vi "ReadWrite Label.vi"(5 "Mode":T13, 6 "ScheduledSDI":bool, 7 "Iteration":i32, 8 "error in (no error)":errorcluster, 10 "FIFOs In":T1, 11 "Label In":T2 {"Words"."Param Setting"."Num Bits" min=1 max=32; "Words"."Param Setting"."Start Bit" min=8 max=31; "Words"."Block Data Refs"."Data Reference" format="%.0x"; "Label" format="%.0o"}) -> (0 "error out":errorcluster, 2 "FIFOs Out":T1, 3 "Label Out":T2 {"Words"."Param Setting"."Num Bits" min=1 max=32; "Words"."Param Setting"."Start Bit" min=8 max=31; "Words"."Block Data Refs"."Data Reference" format="%.0x"; "Label" format="%.0o"})   [LabVIEW 2012, in "AIT 429 Custom Device.lvlib"]
uses:
  AIT 429 Custom Device.lvlib
  RT Controls/ReadWrite Selector.ctl
  Controls and Global/Label.ctl
  Controls and Global/transferPeriod.ctl
  <vilib>/NI Veristand/Custom Device API/Data Reference.ctl
  <vilib>/NI Veristand/Custom Device API/Custom Device API.lvlib
  <vilib>/NI Veristand/Custom Device API/Block Data Reference.ctl
  Controls and Global/Start Bit.ctl
  Controls and Global/Number of Bits.ctl
  RT Controls/RT Label Settings.ctl
  RT Controls/FIFO.ctl
  RT Controls/Driver Data.ctl
  RT Controls/RT Param Setting.ctl
  RT Controls/RT Word Settings.ctl
  Controls and Global/TransferType.ctl
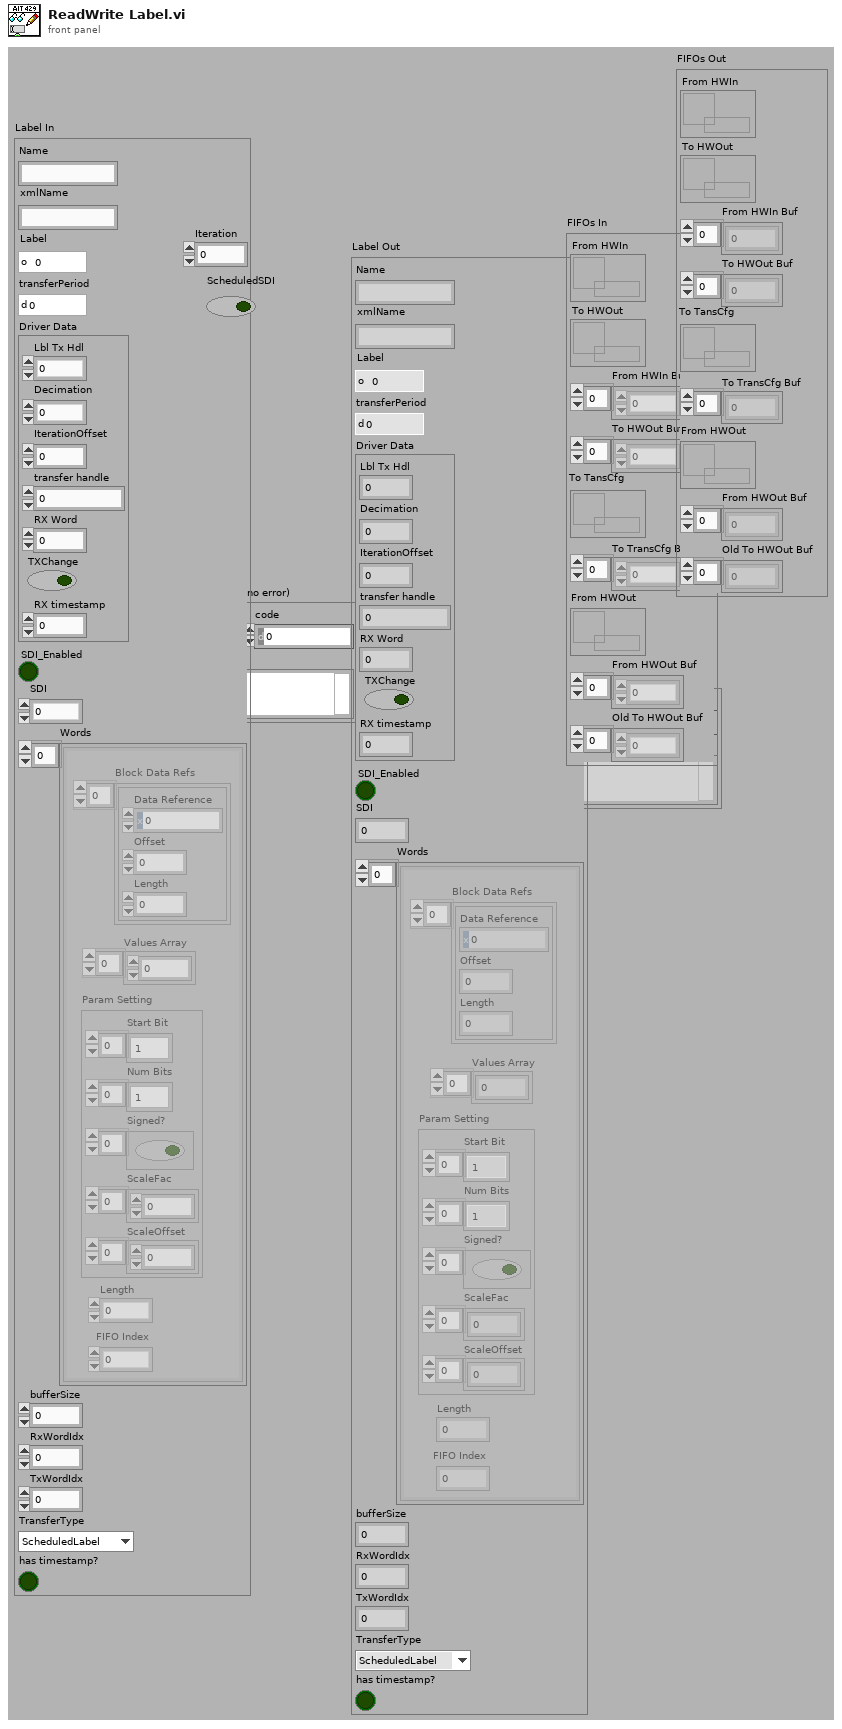
[diagram p1: front panel]
types:
  T1 = typedef "AIT 429 Custom Device.lvlib/FIFO.ctl" = cluster{"From HWIn":refnum<k33>, "To HWOut":refnum<k33>, "From HWIn Buf":dbl[], "To HWOut Buf":dbl[], "To TansCfg":refnum<k33>, "To TransCfg Buf":dbl[], "From HWOut":refnum<k33>, "From HWOut Buf":dbl[], "Old To HWOut Buf":dbl[]}
  T2 = typedef "AIT 429 Custom Device.lvlib/RT Label Settings.ctl" = cluster{"Name":string, "xmlName":string, "Label":T3, "transferPeriod":T4, "Driver Data":T5, "SDI_Enabled":bool, "SDI":u8, "Words":T6[], "bufferSize":u32, "RxWordIdx":i32, "TxWordIdx":i32, "TransferType":T12, "has timestamp?":bool}
  T3 = typedef "AIT 429 Custom Device.lvlib/Label.ctl" = u8
  T4 = typedef "AIT 429 Custom Device.lvlib/transferPeriod.ctl" = u32
  T5 = typedef "AIT 429 Custom Device.lvlib/Driver Data.ctl" = cluster{"Lbl Tx Hdl":u32, "Decimation":i32, "IterationOffset":i32, "transfer handle":u32, "RX Word":u32, "TXChange":bool, "RX timestamp":dbl}
  T6 = typedef "AIT 429 Custom Device.lvlib/RT Word Settings.ctl" = cluster{"Block Data Refs":T7[], "Values Array":dbl[], "Length":i32, "FIFO Index":i32, "Param Setting":T9}
  T7 = typedef "Custom Device API.lvlib/Block Data Reference.ctl" = cluster{"Data Reference":T8, "Offset":i32, "Length":i32}
  T8 = typedef "Custom Device API.lvlib/Data Reference.ctl" = i32
  T9 = typedef "AIT 429 Custom Device.lvlib/Rt Param Setting.ctl" = cluster{"Start Bit":T10[], "Num Bits":T11[], "Signed?":bool[], "ScaleFac":dbl[], "ScaleOffset":dbl[]}
  T10 = typedef "AIT 429 Custom Device.lvlib/Start Bit.ctl" = i32
  T11 = typedef "AIT 429 Custom Device.lvlib/Number of Bits.ctl" = i32
  T12 = typedef "AIT 429 Custom Device.lvlib/TransferType.ctl" = enum16{"ScheduledLabel", "Acyclic", "Block", "Strobe"}
  T13 = typedef "AIT 429 Custom Device.lvlib/ReadWrite Selector.ctl" = enum16{"Inline Read", "Inline Write", "Async HWIn", "Async HWOut"}
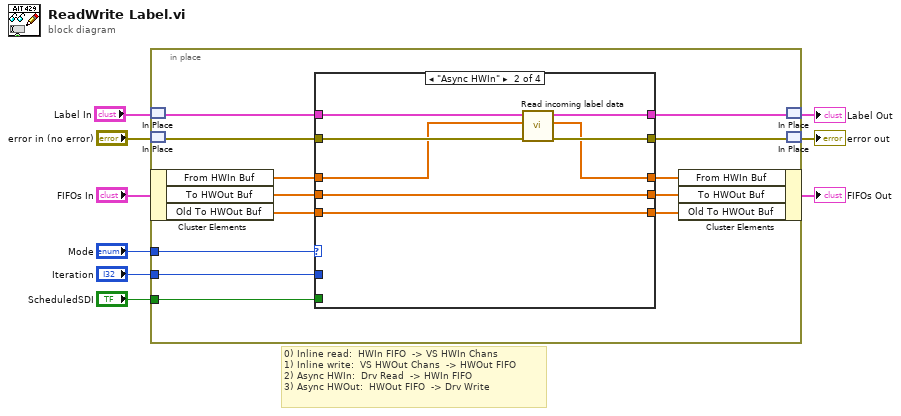
[diagram p0: block diagram]
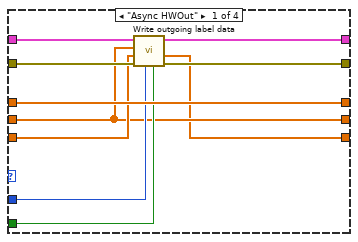
[diagram p2: hidden frame]
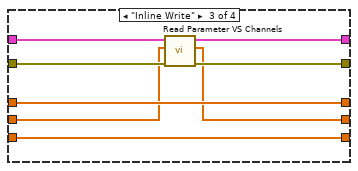
[diagram p3: hidden frame]
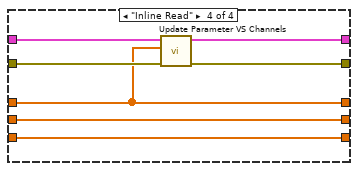
[diagram p4: hidden frame]
diagram:
  # "0) Inline read:\t\tHWIn FIFO \t-> VS HWIn Chans\n1) Inline write: \tVS HWOut Chans \t-> HWOut FIFO\n2) Async HWIn:\t\tDrv Read \t-> HWIn FIFO\n3) Async HWOut: \tHWOut FIFO \t-> Drv Write"
  n1 = in-place {
    in-place-border: "Mode" -> [w14]
    in-place-border: "Iteration" -> [w16]
    in-place-border: "ScheduledSDI" -> [w15]
    n2 = in-place-match #1("Label In") -> (w13:T2)
    n3 = in-place-match #2("error in (no error)") -> (w21:errorcluster)
    n4 = in-place-cluster #3("FIFOs In") -> ("From HWIn Buf"=w17:dbl[], "To HWOut Buf"=w18:dbl[], "Old To HWOut Buf"=w11:dbl[])
    n5 = case shown="\"Async HWIn\"" w14 {
      tunnel: [w32 w40 w48 w55] -> w22
      tunnel: w21 -> [w31 w39 w47 w54]
      tunnel: [w24 w38 w45 w53] -> w20
      tunnel: [w30 w34 w46 w52] -> w19
      tunnel: w18 -> [w24 w38 w42 w53]
      tunnel: w17 -> [w30 w35 w46 w52]
      tunnel: w16 -> [w29 _ _ _]
      tunnel: w15 -> [w28 _ _ _]
      tunnel: w11 -> [w25 w33 w41 w49]
      tunnel: w13 -> [w27 w37 w44 w51]
      tunnel: [w26 w36 w43 w50] -> w12
      tunnel: [w23 w33 w41 w49] -> w10
      frame "Async HWOut" {
        n6 = call "Write outgoing label data.vi"("ScheduledSDI"=w28, "Iteration"=w29, "error in (no error)"=w31, "Last iteration values"=w25, "This iteration values"=w24, "Label Settings"=w27) -> ("error out"=w32:errorcluster, "Last iteration values Out"=w23:dbl[], "Label Settings"=w26:T2)  [unwired: 3 in]
      }
      frame "Async HWIn" {
        n7 = call "Read incoming label data.vi"("error in (no error)"=w39, "From HWIn Buf in"=w35, "Label Settings"=w37) -> ("error out"=w40:errorcluster, "From HWIn Buf out"=w34:dbl[], "Label Settings Out"=w36:T2)  [unwired: 6 in]
      }
      frame "Inline Write" {
        n8 = call "Read Parameter VS Channels.vi"("error in (no error)"=w47, "To HWOut Buf in"=w42, "Label Settings"=w44) -> ("error out"=w48:errorcluster, "To HWOut Buf out"=w45:dbl[], "Label Settings"=w43:T2)  [unwired: 6 in]
      }
      frame "Inline Read" {
        n9 = call "Update Parameter VS Channels.vi"("error in (no error)"=w54, "From HWIn Buf"=w52, "Label Settings"=w51) -> ("error out"=w55:errorcluster, "Label Settings"=w50:T2)  [unwired: 7 in]
      }
    }
    n10 = in-place-cluster #3("From HWIn Buf"=w19, "To HWOut Buf"=w20, "Old To HWOut Buf"=w10) -> (→"FIFOs Out":T1)
    n11 = in-place-match #1(w12) -> (→"Label Out":T2)
    n12 = in-place-match #2(w22) -> (→"error out":errorcluster)
  }
